vi "P2018 TB INCAR_Change.vi"(9 "error in (no error)":errorcluster, 10 "Change":T1) -> (1 "error out":errorcluster, 2 "Change?":T1)   [LabVIEW 2013]
uses:
  Controles/Change Control.ctl
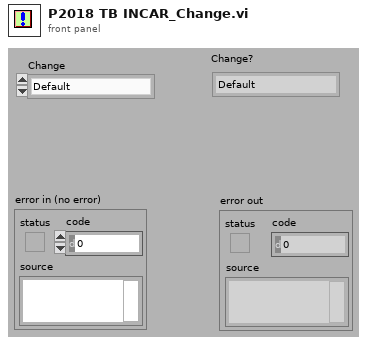
[diagram p1: front panel]
types:
  T1 = typedef "Change Control.ctl" = enum16{"Default", "Continue", "Change Flows", "Change Valves", "Change Temp"}
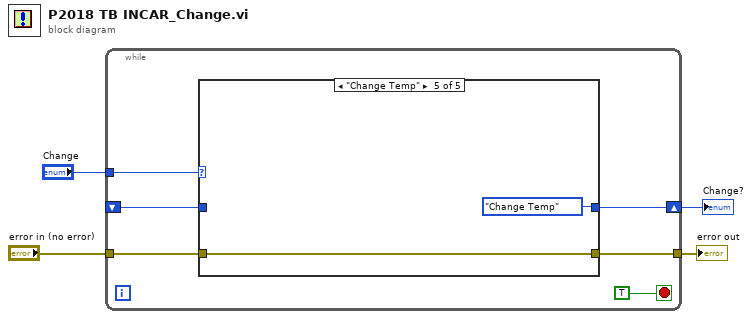
[diagram p0: block diagram]
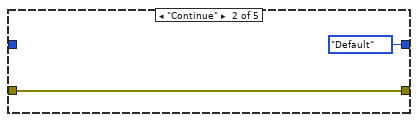
[diagram p3: hidden frame]
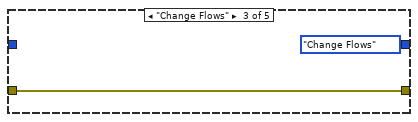
[diagram p4: hidden frame]
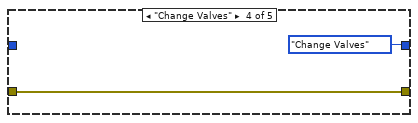
[diagram p5: hidden frame]
diagram:
  n1 = while {
    tunnel: "Change" -> [w10]
    shift-right: [w8] -> w3
    shift-left: _ -> [w7]
    tunnel: "error in (no error)" -> [w6]
    tunnel: [w5] -> w1
    stop <- TRUE stop-if-true
    n2 = case shown="\"Change Temp\"" w10 {
      tunnel: [w12 Change_Control."Default" ("Change 2") Change_Control."Change Flows" ("Change 2") Change_Control."Change Valves" ("Change 2") Change_Control."Change Temp" ("Change 2")] -> w8
      tunnel: w7 -> [w12 _ _ _ _]
      tunnel: w6 -> [w11 w14 w16 w18 w20]
      tunnel: [w11 w14 w16 w18 w20] -> w5
      frame "Default", Default {
      }
      frame "Continue" {
      }
      frame "Change Flows" {
      }
      frame "Change Valves" {
      }
      frame "Change Temp" {
      }
    }
  }
  "Change?" <- w3
  "error out" <- w1
